vi "Run.vi"(8 "error in (no error)":errorcluster, 11 "FormulaLV App in":refnum<class "FormulaG App.lvclass">) -> (0 "error out":errorcluster, 3 "FormulaLV App out":refnum<class "FormulaG App.lvclass">)   [LabVIEW 2020, in "FormulaG.lvlib" / "FormulaG App.lvclass"]
uses:
  FormulaG App.lvclass
  FormulaG App.lvclass/FormulaG App.ctl
  <vilib>/IlluminatedG/IG HTTP Server/HTTP Server/Server/Server.lvclass
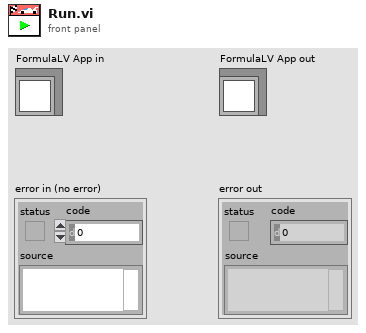
[diagram p1: front panel]
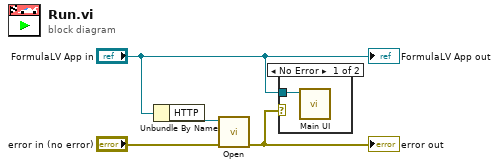
[diagram p0: block diagram]
diagram:
  n1 = Unbundle By Name("FormulaLV App in") -> ("HTTP"=w3:refnum<class "Server.lvclass">)
  n2 = call <vilib>:"Open.vi"("error in (no error)"="error in (no error)", "Server in"=w3) -> ("error out"=w1:errorcluster)  [unwired: 8 in, 1 out]
  "error out" <- w1
  n3 = case shown="No Error" w1 {
    tunnel: "FormulaLV App in" -> [w5 _]
    frame No Error {
      n4 = call "Main UI.vi"("FormulaLV App in"=w5) -> ()  [unwired: 11 in]
    }
    frame Error {
    }
  }
  "FormulaLV App out" <- "FormulaLV App in"
